vi "Read Instance.vi"(11 "Dependency in":refnum<class "Dependency.lvclass">) -> (2 "SMO.lvclass":refnum<class "SMO.lvclass">, 3 "Dependency out":refnum<class "Dependency.lvclass">)   [LabVIEW 2021, in "smo.lvlib" / "Dependency.lvclass"]
uses:
  Dependency.lvclass
  SMO/SMO.lvclass
  Dependency.lvclass/Dependency.ctl
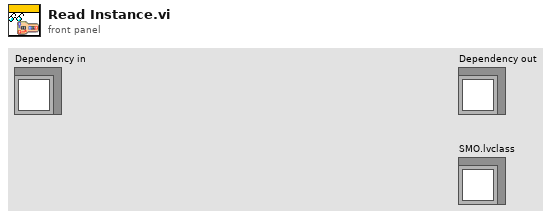
[diagram p1: front panel]
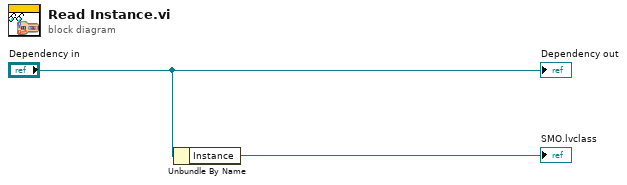
[diagram p0: block diagram]
diagram:
  n1 = Unbundle By Name("Dependency in") -> ("Instance"=→"SMO.lvclass":refnum<class "SMO.lvclass">)
  "Dependency out" <- "Dependency in"
